vi "Get aperture images.vi"(8 "error in (no error)":errorcluster caption="错误输入（无错误）", 10 "Image Name":string="I1", 11 "ParamsUI":T2={"IsNorImage"=TRUE, "Exposure Values"=100289, "ImagePath"=path "C:/Users/hedongpo/Desktop/514-hdp/Alignment Assemble System/Test Picture/B/3.bmp"} caption="参数界面" {"Exposure Values" scale=0.0..200000.0}) -> (0 "error out":errorcluster caption="错误输出", 2 "Session Out":T1, 3 "Image out":T3(plugin-control), 4 "数值":dbl)   [LabVIEW 2017]
uses:
  <vilib>/userdefined/High Color/IMAQdx.ctl
  <vilib>/vision/driver/IMAQdx.llb/IMAQdx Buffer Number Mode.ctl
  Global System.vi
  <resource>/objmgr/imaqdx.rc
  <vilib>/vision/driver/NI_Vision_Acquisition_Software.lvlib
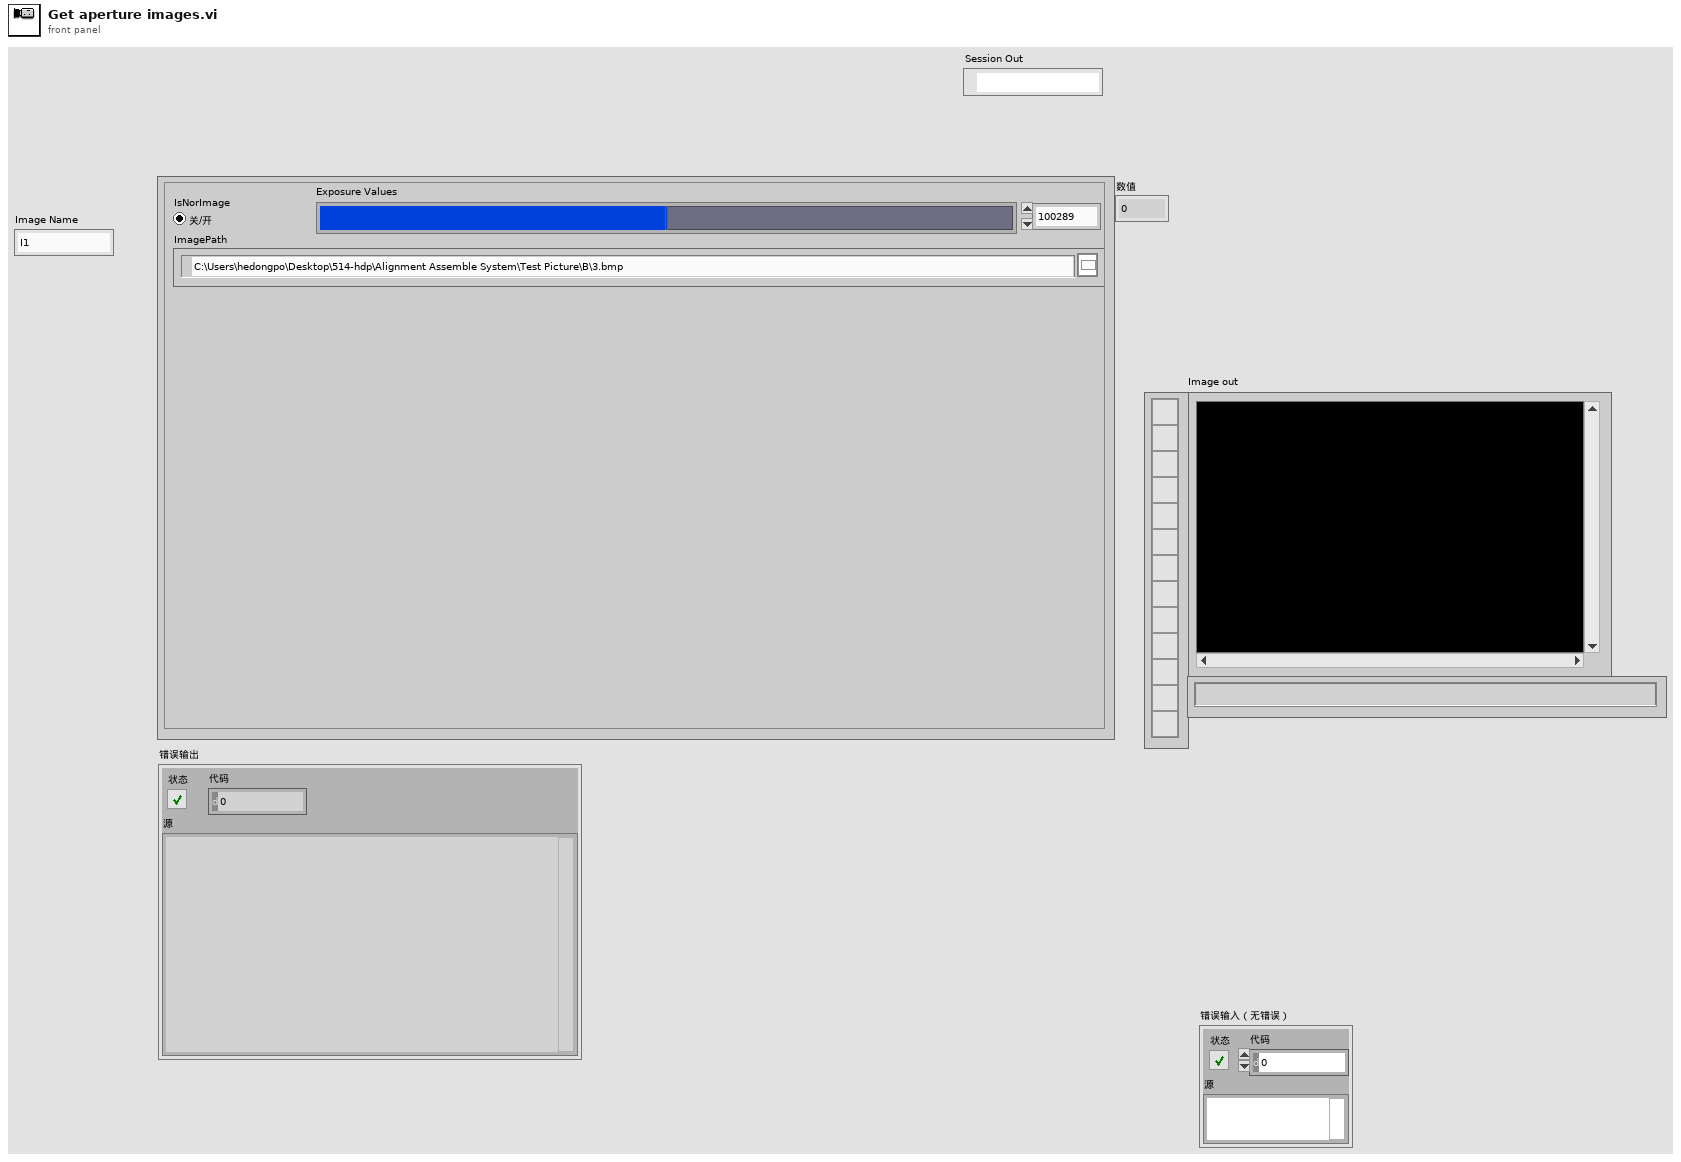
[diagram p1: front panel]
types:
  T1 = typedef "IMAQdx.ctl" = refnum<k21>
  T2 = cluster{"IsNorImage":bool, "Exposure Values":i64, "ImagePath":path}
  T3 = typedef "IMAQ Image.ctl" = refnum<image>
  T4 = typedef "Image Type" = u32
  T5 = cluster{"IsNorImage":bool, "Exposure Values":u32, "ImagePath":path}
  T6 = typedef "NI_Vision_Acquisition_Software.lvlib/IMAQdx Buffer Number Mode.ctl" = enum32{"Next", "Last", "Buffer Number", "Every", "Last New"}
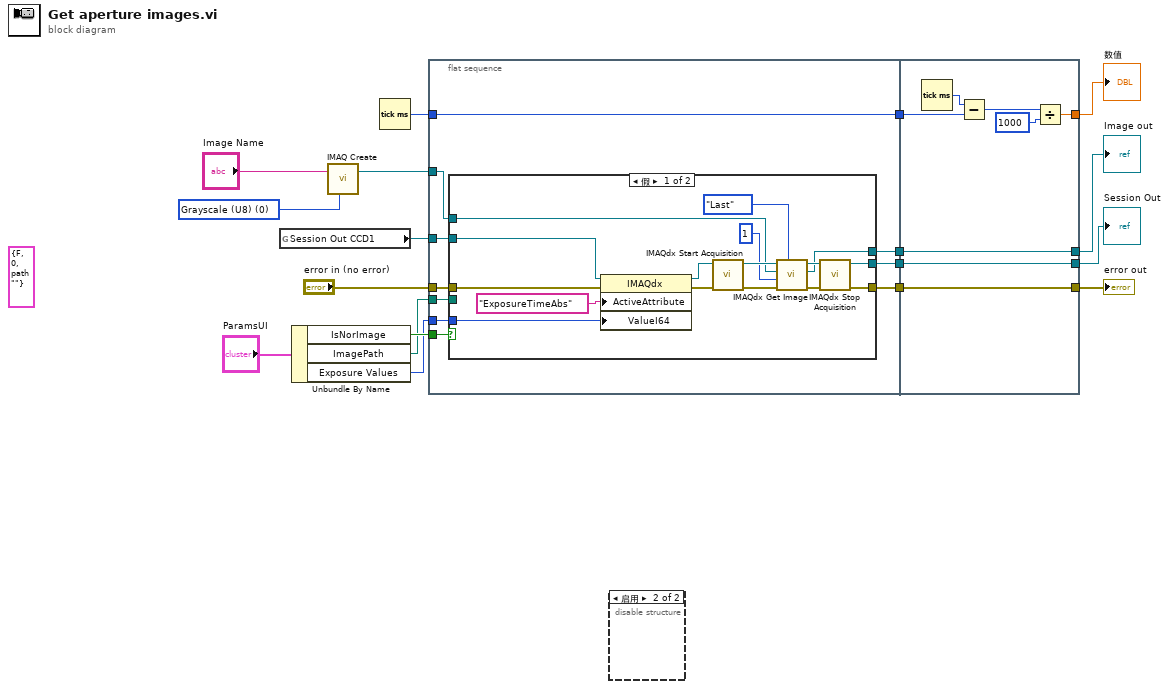
[diagram p0: block diagram]
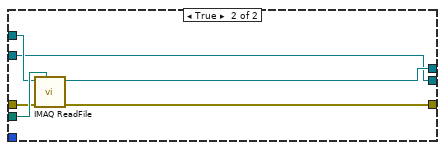
[diagram p2: hidden frame]
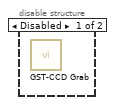
[diagram p3: hidden frame]
diagram:
  w11 = T4 0 items=["Grayscale (U8)", "Grayscale (I16)", "Grayscale (SGL)", "Complex (CSG)", "RGB (U32)", "HSL (U32)", "RGB (U64)", "Grayscale (U16)"] ("Image Type")
  (unwired) T5 {"IsNorImage"=FALSE, "Exposure Values"=0, "ImagePath"=path ""} ("ParamsUI")
  n1 = global read "Global System.vi" "Session Out CCD1"() -> (w8:T1)
  n2 = Unbundle By Name("ParamsUI") -> ("IsNorImage"=w18:bool, "ImagePath"=w17:path, "Exposure Values"=w16:i64)
  n3 = call "IMAQ Create"("Image Name"="Image Name", "Image Type"=w11) -> ("New Image"=w14:T3)  [unwired: 3 in, 1 out]
  n4 = Tick Count (ms)() -> (millisecond timer value=w6:u32)
  n5 = flat-sequence {
    tunnel: w18 -> [w28]
    tunnel: w17 -> [w27]
    tunnel: w16 -> [w26]
    tunnel: w14 -> [w25]
    tunnel: "error in (no error)" -> [w24]
    tunnel: w8 -> [w21]
    tunnel: w6 -> [w19]
    tunnel: [w23] -> w5
    tunnel: [w22] -> w4
    tunnel: [w20] -> w3
    tunnel: [w19] -> w2
    tunnel: [w56] -> w7
    tunnel: [w57] -> w9
    tunnel: [w58] -> w12
    tunnel: w5 -> [w58]
    tunnel: w4 -> [w57]
    tunnel: w3 -> [w56]
    tunnel: w2 -> [w54]
    tunnel: [w51] -> w1
    frame #0 {
      n6 = case shown="假" w28 {
        tunnel: w27 -> [_ w50]
        tunnel: [w29 w49] -> w22
        tunnel: w26 -> [w34 _]
        tunnel: w21 -> [w36 w45]
        tunnel: w25 -> [w39 w48]
        tunnel: w24 -> [w35 w47]
        tunnel: [w37 w46] -> w23
        tunnel: [w38 w45] -> w20
        frame False {
          n7 = property class="IMAQdx"(reference=w36, error in=w35, "ActiveAttribute"="ExposureTimeAbs", "ValueI64"=w34) -> (reference out=w33:T1, error out=w32:errorcluster)
          n8 = call <vilib>:"IMAQdx Start Acquisition.vi"("error in"=w32, "Session In"=w33) -> ("error out"=w43:errorcluster, "Session Out"=w44:T1)  [unwired: 8 in]
          n9 = call <vilib>:"IMAQdx Get Image.vi"("Buffer Number Mode (Next)"=IMAQdx_Buffer_Number_Mode."Last", "error in"=w43, "Buffer Number In"=u32 1, "Image In"=w39, "Session In"=w44) -> ("error out"=w30:errorcluster, "Image Out"=w29:T3, "Session Out"=w40:T1)  [unwired: 3 in, 1 out]
          n10 = call <vilib>:"IMAQdx Stop Acquisition.vi"("error in"=w30, "Session In"=w40) -> ("error out"=w37:errorcluster, "Session Out"=w38:T1)  [unwired: 8 in]
        }
        frame True {
          n11 = call "IMAQ ReadFile"("File Path"=w50, "error in (no error)"=w47, "Image"=w48) -> ("error out"=w46:errorcluster, "Image Out"=w49:T3)  [unwired: 4 in, 3 out]
        }
      }
    }
    frame #1 {
      n12 = Tick Count (ms)() -> (millisecond timer value=w55:u32)
      n13 = Subtract(x=w55, y=w54) -> (x-y=w53:u32)
      n14 = Divide(x=w53, y=u32 1000) -> (x/y=w51:dbl)
    }
  }
  n15 = disable-structure shown="启用" {
    frame Disabled {
      n16 = call "GST-CCD Grab.vi"() -> ()  [unwired: 9 in, 3 out]
    }
    frame Enabled {
    }
  }
  "Image out" <- w9
  "error out" <- w12
  "Session Out" <- w7
  "数值" <- w1
